vi "Add Key-Value Pair.vi"(8 "error in (no error)":errorcluster, 11 "URI in":refnum<class "URI.lvclass">) -> (0 "error out":errorcluster, 3 "URI out":refnum<class "URI.lvclass">)   [LabVIEW 2013, in "openURI.lvlib" / "URI.lvclass"]
uses:
  URI.lvclass
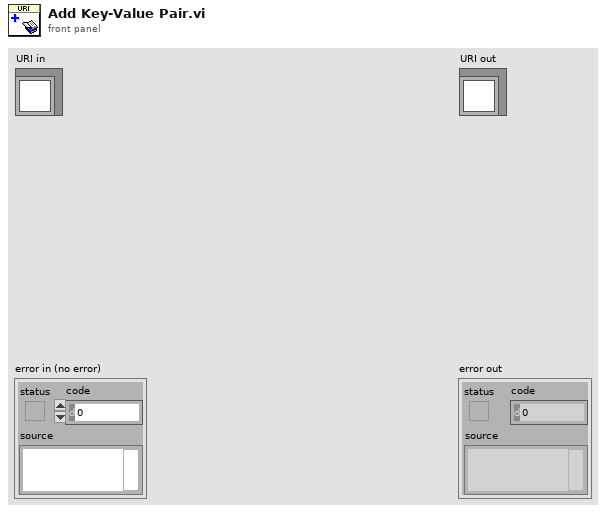
[diagram p1: front panel]
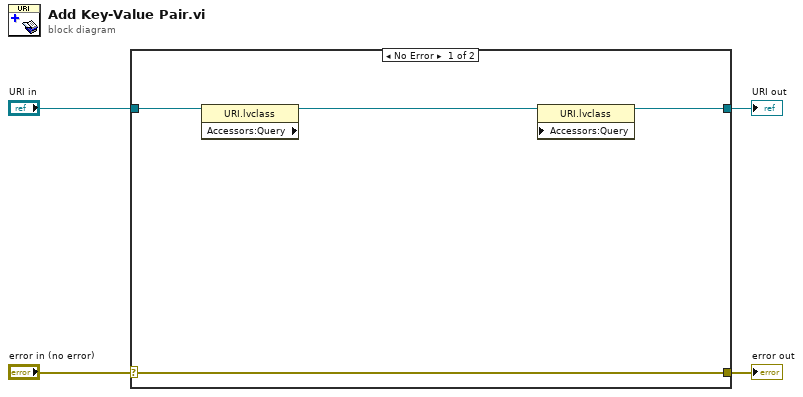
[diagram p0: block diagram]
diagram:
  n1 = case shown="No Error" "error in (no error)" {
    selector: "error in (no error)" -> [w8 w10]
    tunnel: [w8 w10] -> w3
    tunnel: [w5 w9] -> w1
    tunnel: "URI in" -> [w7 w9]
    frame No Error {
      n2 = property class="URI.lvclass" props=["Accessors:Query"](reference=w7) -> (reference out=w6:refnum<class "URI.lvclass">)  [unwired: 1 in, 2 out]
      n3 = property class="URI.lvclass" props=["Accessors:Query"](reference=w6) -> (reference out=w5:refnum<class "URI.lvclass">)  [unwired: 2 in, 1 out]
    }
    frame Error {
    }
  }
  "error out" <- w3
  "URI out" <- w1
